vi "Randomise String.vi"(11 "String in":string) -> (3 "String out":string)   [LabVIEW 2018, in "Create New Assert Tester.lvclass"]
uses:
  Create New Assert Tester.lvclass
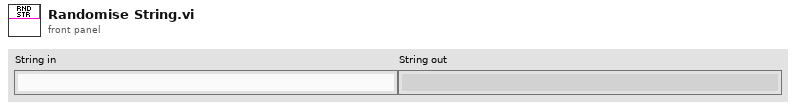
[diagram p1: front panel]
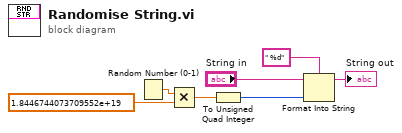
[diagram p0: block diagram]
diagram:
  n1 = Random Number (0-1)() -> (number: 0 to 1=w7:dbl)
  n2 = Multiply(x=w7, y=1.8446744073709552e+19 ("I8 Comparison Value 2")) -> (x*y=w5:dbl)
  n3 = To Unsigned Quad Integer(1:w5) -> (0:w4:u64)
  n4 = Format Into String(format string=" %d", initial string="String in", w4) -> (resulting string=→"String out":string)  [unwired: 1 in, 1 out]
